vi "Periodic Tasks.vi"(8 "error in":errorcluster) -> ()   [LabVIEW 2014]
doc: "This VI runs in parallel to other tasks. It can contain as many user-defined periodic loops as you need. These can carry out PID or other sorts of timed response."
uses:
  <vilib>/Rock Robotics/WPI/Solenoid/WPI_SolenoidValue.ctl
  teleop_autoFeed.ctl
  <vilib>/Rock Robotics/WPI/CAN/TalonSRX/WPI_CANTalonSRX_APIControlMode.ctl
  <vilib>/Rock Robotics/WPI/CAN/TalonSRX/WPI_CANTalonSRX_Params.ctl
  Robot Global Data.vi
  <vilib>/Rock Robotics/WPI/Solenoid/WPI_SolenoidSetEnum.vi
  <vilib>/Rock Robotics/Network Tables/SD Write Number.vi
  <vilib>/Rock Robotics/WPI/RobotDrive/WPI_RobotDriveGetSetRefNum.vi
  <vilib>/Rock Robotics/WPI/Joystick/WPI_JoystickGetSetRefNum.vi
  <vilib>/Rock Robotics/Network Tables/SD Read Boolean.vi
  <vilib>/Rock Robotics/WPI/RobotDrive/WPI_RobotDriveArcadeDrive_Standard(NoSaturation).vi
  <vilib>/addons/control/pid/pid.llb/PID (DBL).vi
  <vilib>/addons/control/pid/NI_PID_pid.lvlib
panel:
  out "Distance":dbl
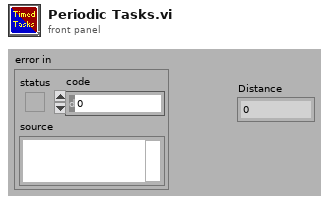
[diagram p1: front panel]
types:
  T1 = typedef "teleop_autoFeed.ctl" = enum16{"wait", "initialize", "arms down 1", "arms open", "arms down 2", "arms close", "up 1st", "back/up"}
  T2 = typedef "WPI_SolenoidValue.ctl" = enum16{"Off", "On", "Forward", "Reverse"}
  T3 = typedef "WPI_SolenoidDevRef.ctl" = cluster{"DevStatus":errorcluster, "Pneumatics Control Module":u8, "Forward Solenoid Channel":T4, "Reverse Solenoid Channel":T4}
  T4 = typedef "WPI_SolenoidChannel.ctl" = enum8{"Solenoid 0", "Solenoid 1", "Solenoid 2", "Solenoid 3", "Solenoid 4", "Solenoid 5", "Solenoid 6", "Solenoid 7", "Invalid"}
  T5 = typedef "WPI_MotorControlDeviceRef.ctl" = cluster{"DeviceStatus":errorcluster, "Type":T6, "PWM":cluster{"Controller":T7, "PWM Channel":T8, "DeadBand":T9}, "CAN":cluster{"Device Number":u8, "Control Mode":T10, "Semaphore":T11, "Max Vout":dbl, "TalonSRX Control Mode":T12}, "Invert":bool, "TransformRef":T13, "InvTransformRef":T13}
  T6 = typedef "WPI_MotorControlType.ctl" = enum16{"PWM", "CAN", "CANTalonSRX"}
  T7 = typedef "FPGA_TypedefDigitalModule.ctl" = enum16{"Controller 1"}
  T8 = typedef "FPGA_DIOPWMChannel.ctl" = enum8{"PWM 0", "PWM 1", "PWM 2", "PWM 3", "PWM 4", "PWM 5", "PWM 6", "PWM 7", "PWM 8", "PWM 9", "PWM MXP 0", "PWM MXP 1", "PWM MXP 2", "PWM MXP 3", "PWM MXP 4", "PWM MXP 5", "PWM MXP 6", "PWM MXP 7", "PWM MXP 8", "PWM MXP 9", "Invalid"}
  T9 = typedef "WPI_PWMDeadband.ctl" = cluster{"Name":string, "maxPositivePwm":i32, "minPositivePwm":i32, "centerPwm":i32, "maxNegativePwm":i32, "minNegativePwm":i32, "angularRange":u16}
  T10 = typedef "WPI_CANJaguar_ControlMode.ctl" = enum8{"Percent VBus", "Current", "Speed", "Position", "Voltage"}
  T11 = typedef "Semaphore RefNum" = refnum<k1>
  T12 = typedef "WPI_CANTalonSRX_APIControlMode.ctl" = enum8{"Percent VBus", "Speed", "Position", "Slave", "Unchanged / Invalid"}
  T13 = typedef "WPI_PWMTransform_ConPane.ctl" = refnum<vi>
  T14 = typedef "WPI_AnalogChannelDevRef.ctl" = cluster{"DevStatus":errorcluster, "Controller":T15, "Analog Channel":T16}
  T15 = typedef "FPGA_TypedefAnalogModule.ctl" = enum16{"Controller 1"}
  T16 = typedef "FPGA_AIChannel.ctl" = enum8{"AI 0", "AI 1", "AI 2", "AI 3", "AI MXP 0", "AI MXP 1", "AI MXP 2", "AI MXP 3", "Invalid"}
  T17 = typedef "WPI_CANTalonSRX_GlobalStatus.ctl" = cluster{"Applied Throttle":dbl, "Module Enabled":bool, "CAN Error":errorcluster, "Closed Loop Error":dbl, "Forward Limit Switch Closed":bool, "Reverse Limit Switch Closed":bool, "Sensor Position":dbl, "Sensor Velocity":dbl, "Current":dbl, "Sticky Fault - Over Temp":bool, "Sticky Fault - Under Voltage":bool, "Sticky Fault - Forward Limit":bool, "Sticky Fault - Reverse Limit":bool, "Sticky Fault - Forward Soft Limit":bool, "Sticky Fault - Reverse Soft Limit":bool, "Brake is Enabled":bool, "Encoder Position":dbl, "Encoder Velocity":dbl, "Encoder Index Count":dbl, "Encoder A Pin State":bool, "Encoder B Pin State":bool, "Encoder Index Pin State":bool, "Analog In":dbl, "Analog In Velocity":dbl, "Temperature (C)":dbl, "Battery Voltage":dbl}
  T18 = typedef "WPI_CANTalonSRX_Params.ctl" = u8
  T19 = typedef "WPI_JoystickDevRef.ctl" = cluster{"Device":T20}
  T20 = typedef "WPI_JoystickDeviceEnum.ctl" = enum16{"USB 0", "USB 1", "USB 2", "USB 3", "USB 4", "USB 5"}
  T21 = typedef "WPI_EncoderDevRef.ctl" = cluster{"DevStatus":errorcluster, "EncoderIndex":T22, "CounterIndex":T23, "DistancePerCount":dbl, "Decoding Type":T24}
  T22 = typedef "FPGA_EncoderIdx.ctl" = enum8{"Enc 0", "Enc 1", "Enc 2", "Enc 3", "Enc 4", "Enc 5", "Enc 6", "Enc 7", "Invalid"}
  T23 = typedef "FPGA_CounterCtrSystemIndex.ctl" = enum8{"Ctr 0", "Ctr 1", "Ctr 2", "Ctr 3", "Ctr 4", "Ctr 5", "Ctr 6", "Ctr 7", "Invalid"}
  T24 = typedef "WPI_EncoderType.ctl" = enum16{"1x", "2x", "4x"}
  T25 = typedef "WPI_RobotDriveDevRef.ctl" = cluster{"DevStatus":errorcluster, "Motors[]":T5[], "Square Inputs":bool, "Max Output":dbl}
  T26 = cluster{"proportional gain (Kc)":dbl, "integral time (Ti, min)":dbl, "derivative time (Td, min)":dbl}
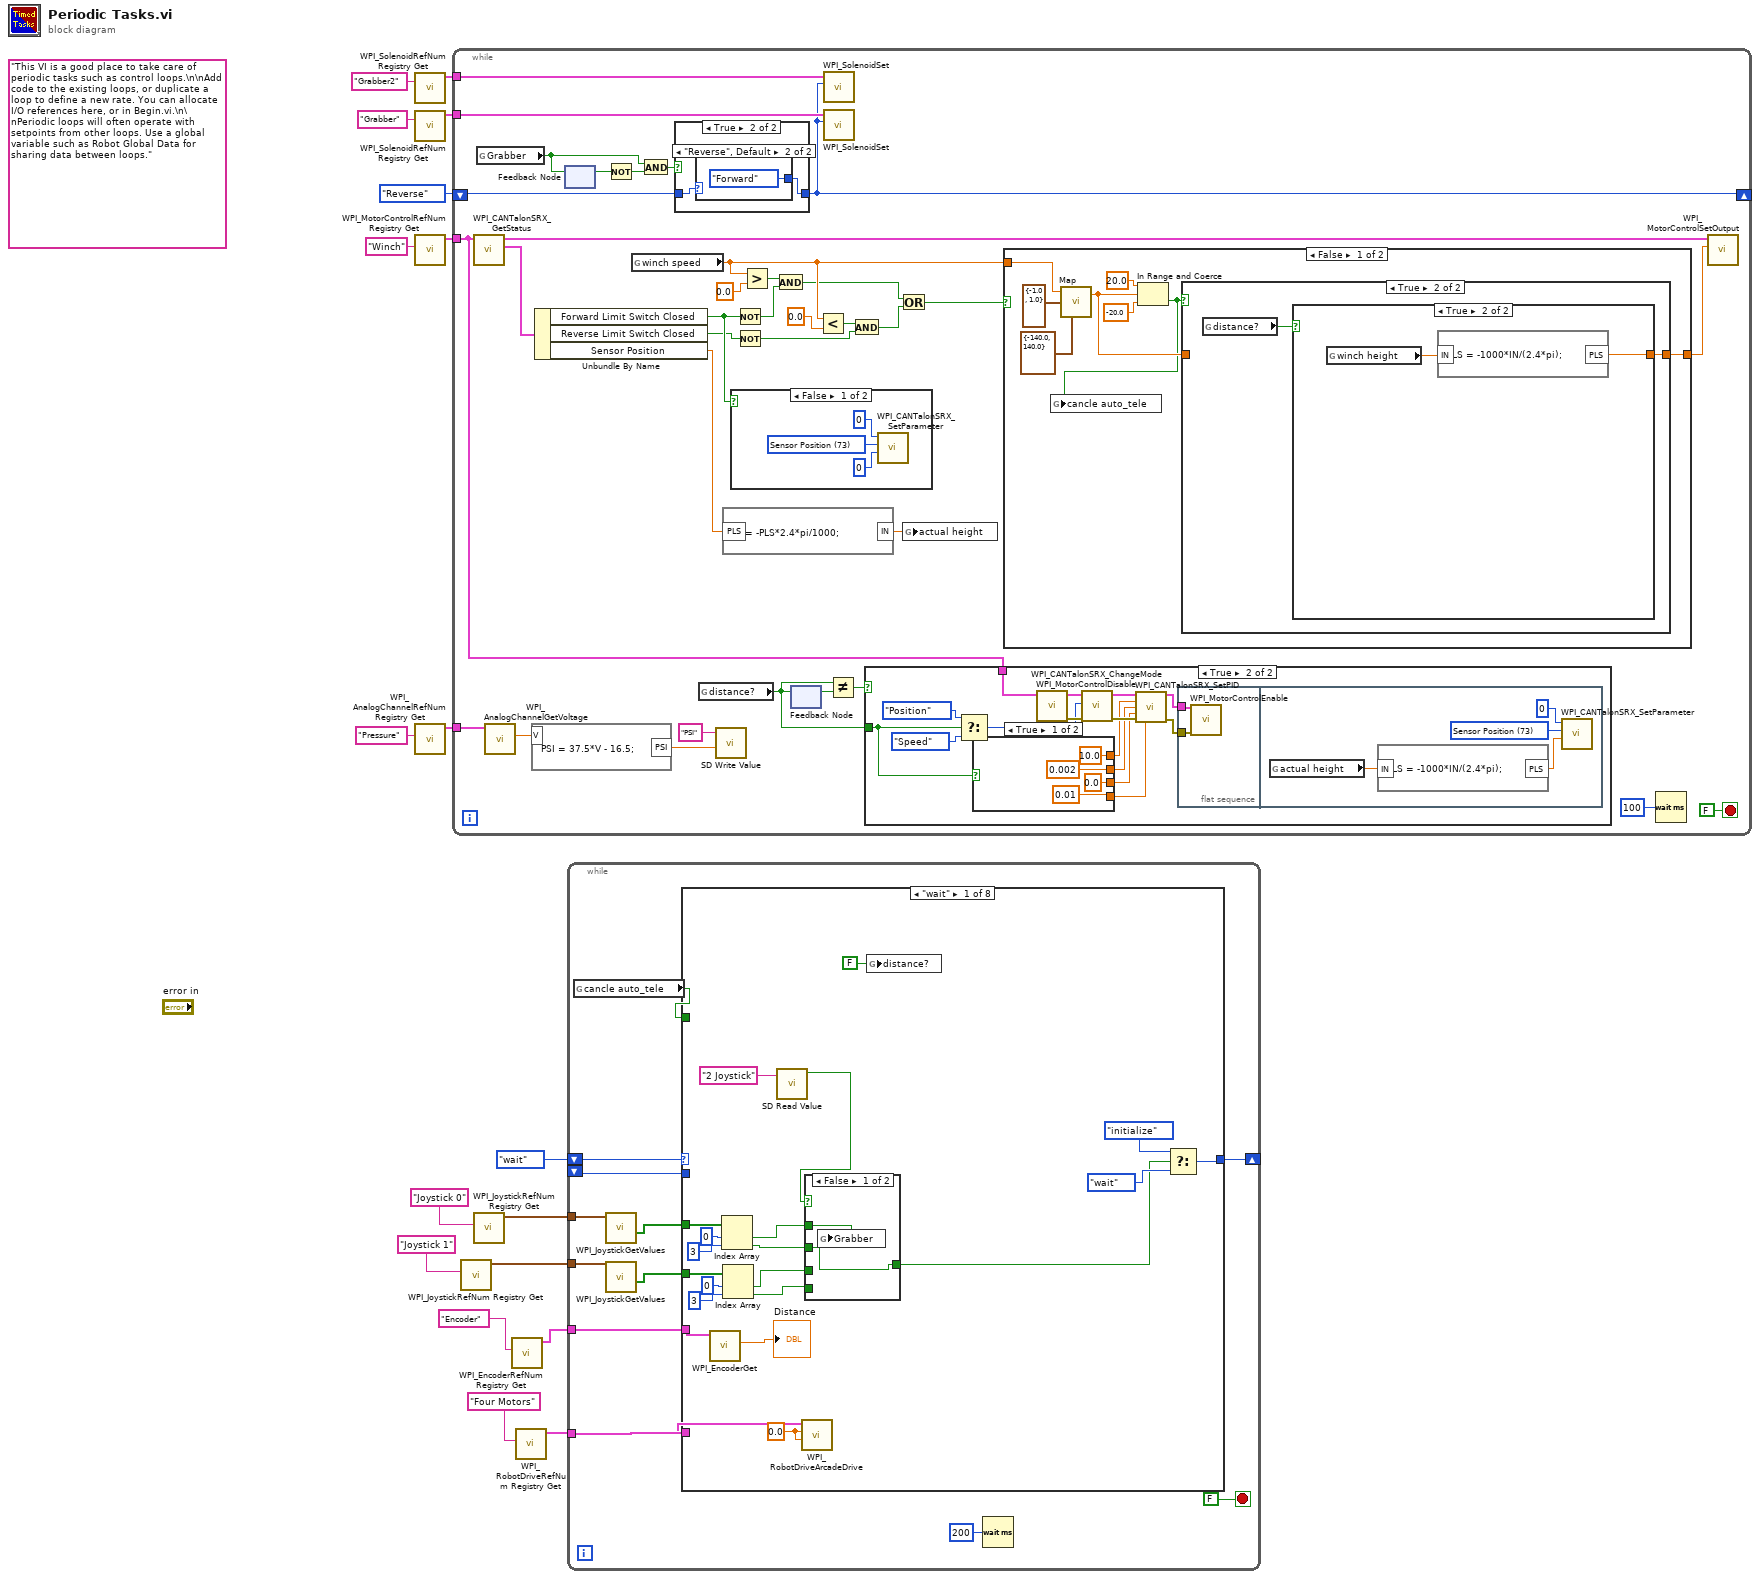
[diagram p0: block diagram]
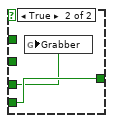
[diagram p2: hidden frame]
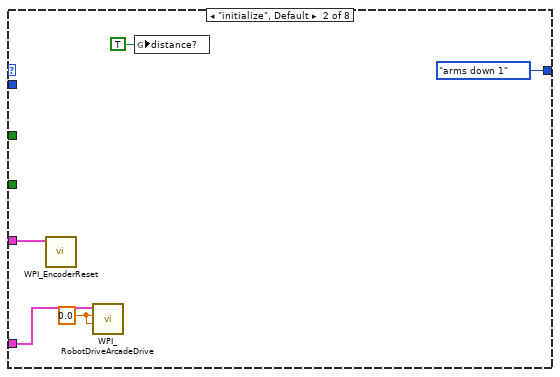
[diagram p3: hidden frame]
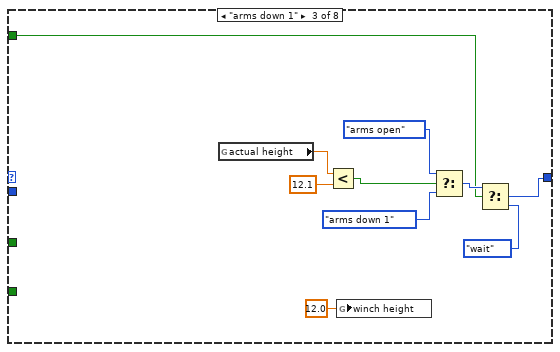
[diagram p4: hidden frame]
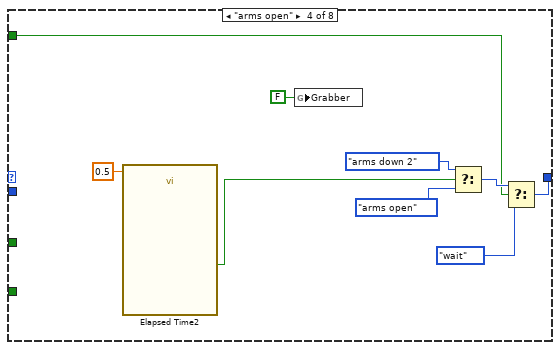
[diagram p5: hidden frame]
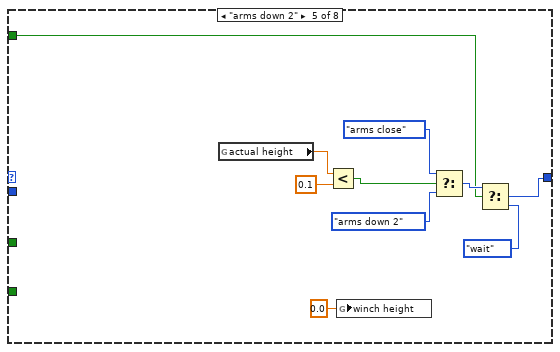
[diagram p6: hidden frame]
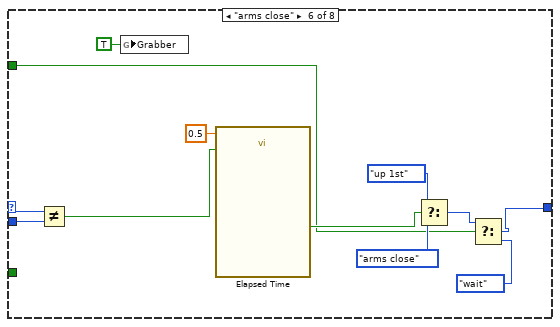
[diagram p7: hidden frame]
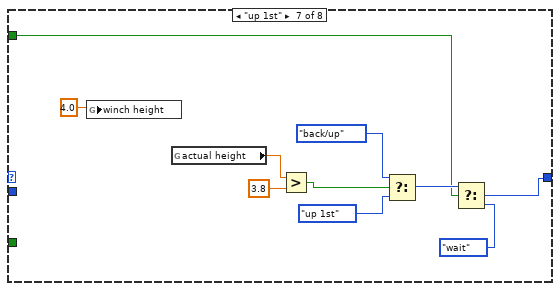
[diagram p8: hidden frame]
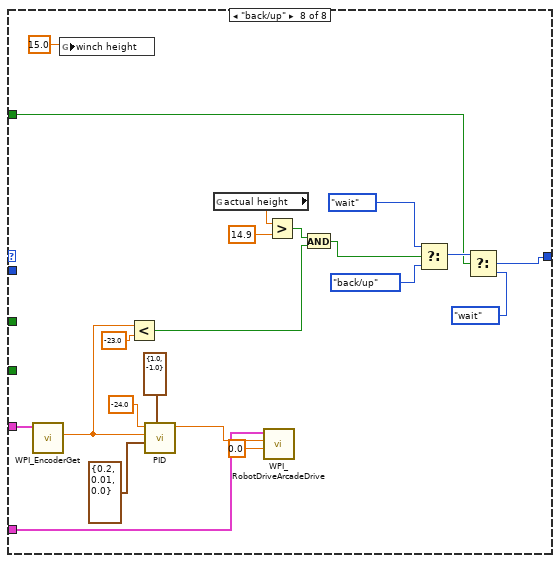
[diagram p9: hidden frame]
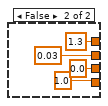
[diagram p11: hidden frame]
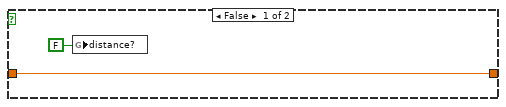
[diagram p13: hidden frame]
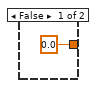
[diagram p14: hidden frame]
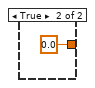
[diagram p15: hidden frame]
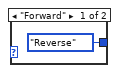
[diagram p17: hidden frame]
diagram:
  w6 = teleop_autoFeed."wait"
  (unwired) "This VI is a good place to take care of periodic tasks such as control loops.\n\nAdd code to the existing loops, or duplicate a loop to define a new rate. You can allocate I/O references here, or in Begin.vi.\n\nPeriodic loops will often operate with setpoints from other loops. Use a global variable such as Robot Global Data for sharing data between loops."
  n1 = call <vilib>:"WPI_SolenoidRefNum Registry Get.vi"("refnum name"="Grabber2") -> ("SolenoidDevRef"=w10:T3)  [unwired: 9 in, 1 out]
  n2 = call <vilib>:"WPI_SolenoidRefNum Registry Get.vi"("refnum name"="Grabber") -> ("SolenoidDevRef"=w16:T3)  [unwired: 9 in, 1 out]
  n3 = call <vilib>:"WPI_MotorControlRefNum Registry Get.vi"("refnum name"="Winch") -> ("MotorControlDevRef"=w14:T5)  [unwired: 9 in, 1 out]
  n4 = call <vilib>:"WPI_AnalogChannelRefNum Registry Get.vi"("refnum name"="Pressure") -> ("AIDeviceRef"=w13:T14)  [unwired: 9 in, 1 out]
  n5 = while {
    tunnel: w16 -> [w48]
    shift-right: [w21] -> _
    shift-left: WPI_SolenoidValue."Reverse" ("Value") -> [w52]
    tunnel: w14 -> [w25]
    tunnel: w13 -> [w44]
    tunnel: w10 -> [w22]
    stop <- FALSE stop-if-true
    n6 = call <vilib>:"WPI_CANTalonSRX_GetStatus.vi"("CAN Talon SRX Ref"=w25) -> ("Talon SRX Status"=w40:T17, "CAN Talon SRX Ref Out"=w29:T5)  [unwired: 8 in, 1 out]
    n7 = global read "Robot Global Data.vi" "Grabber"() -> (w37:bool)
    n8 = call <vilib>:"WPI_AnalogChannelGetVoltage.vi"("AIDeviceRef"=w44) -> ("Voltage"=w47:dbl)  [unwired: 8 in, 2 out]
    n9 = formula code="PSI = 37.5*V - 16.5;"("V"=w47) -> ("PSI"=w46:dbl)
    n10 = Unbundle By Name(w40) -> ("Forward Limit Switch Closed"=w36:bool, "Reverse Limit Switch Closed"=w32:bool, "Sensor Position"=w19:dbl)
    n11 = feedback-in #1(w37) -> ()
    n12 = feedback #1() -> (w49:bool)  [unwired: 1 in]
    n13 = Not(x=w49) -> (.not. x?=w50:bool)
    n14 = global read "Robot Global Data.vi" "winch speed"() -> (w31:dbl)
    n15 = And(x=w37, y=w50) -> (x .and. y?=w51:bool)
    n16 = case shown="True" w51 {
      tunnel: w52 -> [w102 w103]
      tunnel: [w102 w104] -> w21
      frame False {
      }
      frame True {
        n17 = case shown="\"Reverse\", Default" w103 {
          tunnel: [WPI_SolenoidValue."Reverse" ("Value") WPI_SolenoidValue."Forward" ("Value")] -> w104
          frame "Forward" {
          }
          frame "Reverse", Default {
          }
        }
      }
    }
    n18 = global read "Robot Global Data.vi" "distance?"() -> (w26:bool)
    n19 = call-poly <vilib>:"SD Write Value.vi"("Numeric"=w46, "Name"="PSI") -> ()  [unwired: 8 in, 2 out]
    n20 = formula code="IN = -PLS*2.4*pi/1000;"("PLS"=w19) -> ("IN"=w20:dbl)
    n21 = case shown="False" w36 {
      frame False {
        w84 = T18 73 items=["Slot 0 - P"=1, "Slot 0 - I"=2, "Slot 0 - D"=3, "Slot 0 - F"=4, "Slot 0 - I Zone"=5, "Slot 0 - Ramp Rate"=6, "Slot 1 - P"=11, "Slot 1 - I"=12, "Slot 1 - D"=13, "Slot 1 - F"=14, "Slot 1 - I Zone"=15, "Slot 1 - Ramp Rate"=16, "Soft Limit - Forward"=21, "Soft Limit - Reverse"=22, "Soft Limit - Forward Enable"=23, "Soft Limit - Reverse Enable"=24, "On Boot - Brake Mode"=31, "On Boot - Limit Normally Closed - Forward"=32, "On Boot - Limit Normally Closed - Reverse"=33, "On Boot - Limit Disabled - Forward"=34, "On Boot - Limit Disabled - Reverse"=35, "Fault - Over Temp"=41, "Fault - Under Voltage"=42, "Fault - Forward Limit"=43, "Fault - Reverse Limit"=44, "Fault - Hardware Failure"=45, "Fault - Forward Soft Limit"=46, "Fault - Reverse Soft Limit"=47, "Sticky Fault - Over Temp"=48, "Sticky Fault - Under Voltage"=49, "Sticky Fault - Forward Limit"=50, "Sticky Fault - Reverse Limit"=51, "Sticky Fault - Forward Soft Limit"=52, "Sticky Fault - Reverse Soft Limit"=53, "Applied Throttle"=61, "Closed-Loop Error"=62, "Select Feedback Device"=63, "Reverse Closed-Loop Output"=64, "Mode Select"=65, "Profile Slot Select"=66, "Ramp Throttle"=67, "Reverse Feedback Sensor"=68, "Limit Switch Enabled"=69, "Limit Switch Closed - Forward"=70, "Limit Switch Closed - Reverse"=71, "Sensor Position"=73, "Sensor Velocity"=74, "Current"=75, "Brake is Enabled"=76, "Encoder Position"=77, "Encoder Velocity"=78, "Encoder Index Rise Events"=79, "Encoder A Pin State"=80, "Encoder B Pin State"=81, "Encoder Index Pin State"=82, "Analog In with Overflow"=83, "Analog In Velocity"=84, "Temperature"=85, "Battery Voltage"=86, "Reset Count"=87, "Reset Flags"=88, "Firmware Version"=89, "Settings Changed"=90, "Quad Filter Enable"=91, "Ignore Disable Broadcast"=92, "I Accumulator"=93] ("Parameter")
        n22 = call <vilib>:"WPI_CANTalonSRX_SetParameter.vi"("Value"=0, "Parameter"=w84, "Device ID (0)"=u8 0) -> ()  [unwired: 7 in, 2 out]
      }
      frame True {
      }
    }
    n23 = Not(x=w36) -> (.not. x?=w38:bool)
    n24 = Not(x=w32) -> (.not. x?=w35:bool)
    n25 = Greater?(x=w31, y=0.0) -> (0:w39:bool)
    n26 = And(x=w39, y=w38) -> (x .and. y?=w24:bool)
    n27 = feedback-in #2(w26) -> ()
    n28 = feedback #2() -> (w28:bool)  [unwired: 1 in]
    n29 = Less?(x=w31, y=0.0) -> (x < y?=w34:bool)
    n30 = call-poly <vilib>:"WPI_SolenoidSet.vi"("Value"=w21, "SolenoidDevRef"=w22) -> ()  [unwired: 8 in, 2 out]
    n31 = call-poly <vilib>:"WPI_SolenoidSet.vi"("Value"=w21, "SolenoidDevRef"=w48) -> ()  [unwired: 8 in, 2 out]
    n32 = Not Equal?(x=w26, y=w28) -> (x != y?=w27:bool)
    n33 = And(x=w34, y=w35) -> (x .and. y?=w30:bool)
    n34 = case shown="True" w27 {
      tunnel: w26 -> [_ w58]
      tunnel: w25 -> [_ w54]
      frame False {
      }
      frame True {
        n35 = Select(t=WPI_CANTalonSRX_APIControlMode."Position" ("Control Mode"), s=w58, f=WPI_CANTalonSRX_APIControlMode."Speed") -> (s? t:f=w55:T12)
        n36 = case shown="True" w58 {
          tunnel: [10.0 1.3] -> w62
          tunnel: [0.002 0.03] -> w61
          tunnel: [0.0 0.0] -> w60
          tunnel: [0.01 1.0] -> w59
          frame True {
          }
          frame False {
          }
        }
        n37 = call <vilib>:"WPI_MotorControlDisable.vi"("MotorControlDevRef"=w54) -> ("error out"=w57:errorcluster, "MotorControlDevRef"=w56:T5)  [unwired: 9 in]
        n38 = call <vilib>:"WPI_CANTalonSRX_ChangeMode.vi"("error in (no error)"=w57, "Control Mode"=w55, "CAN Talon SRX Ref"=w56) -> ("error out"=w65:errorcluster, "CAN Talon SRX Ref Out"=w66:T5)  [unwired: 7 in]
        n39 = call <vilib>:"WPI_CANTalonSRX_SetPID.vi"("CAN Talon SRX Ref"=w66, "P"=w62, "I"=w61, "D"=w60, "error in (no error)"=w65, "F"=w59) -> ("CAN Talon SRX Ref Out"=w64:T5, "error out"=w63:errorcluster)  [unwired: 8 in]
        n40 = flat-sequence {
          tunnel: w64 -> [w70]
          tunnel: w63 -> [w69]
          frame #0 {
            n41 = call <vilib>:"WPI_MotorControlEnable.vi"("error in (no error)"=w69, "CAN Jaguar Ref"=w70) -> ()  [unwired: 8 in, 2 out]
          }
          frame #1 {
            w72 = T18 73 items=["Slot 0 - P"=1, "Slot 0 - I"=2, "Slot 0 - D"=3, "Slot 0 - F"=4, "Slot 0 - I Zone"=5, "Slot 0 - Ramp Rate"=6, "Slot 1 - P"=11, "Slot 1 - I"=12, "Slot 1 - D"=13, "Slot 1 - F"=14, "Slot 1 - I Zone"=15, "Slot 1 - Ramp Rate"=16, "Soft Limit - Forward"=21, "Soft Limit - Reverse"=22, "Soft Limit - Forward Enable"=23, "Soft Limit - Reverse Enable"=24, "On Boot - Brake Mode"=31, "On Boot - Limit Normally Closed - Forward"=32, "On Boot - Limit Normally Closed - Reverse"=33, "On Boot - Limit Disabled - Forward"=34, "On Boot - Limit Disabled - Reverse"=35, "Fault - Over Temp"=41, "Fault - Under Voltage"=42, "Fault - Forward Limit"=43, "Fault - Reverse Limit"=44, "Fault - Hardware Failure"=45, "Fault - Forward Soft Limit"=46, "Fault - Reverse Soft Limit"=47, "Sticky Fault - Over Temp"=48, "Sticky Fault - Under Voltage"=49, "Sticky Fault - Forward Limit"=50, "Sticky Fault - Reverse Limit"=51, "Sticky Fault - Forward Soft Limit"=52, "Sticky Fault - Reverse Soft Limit"=53, "Applied Throttle"=61, "Closed-Loop Error"=62, "Select Feedback Device"=63, "Reverse Closed-Loop Output"=64, "Mode Select"=65, "Profile Slot Select"=66, "Ramp Throttle"=67, "Reverse Feedback Sensor"=68, "Limit Switch Enabled"=69, "Limit Switch Closed - Forward"=70, "Limit Switch Closed - Reverse"=71, "Sensor Position"=73, "Sensor Velocity"=74, "Current"=75, "Brake is Enabled"=76, "Encoder Position"=77, "Encoder Velocity"=78, "Encoder Index Rise Events"=79, "Encoder A Pin State"=80, "Encoder B Pin State"=81, "Encoder Index Pin State"=82, "Analog In with Overflow"=83, "Analog In Velocity"=84, "Temperature"=85, "Battery Voltage"=86, "Reset Count"=87, "Reset Flags"=88, "Firmware Version"=89, "Settings Changed"=90, "Quad Filter Enable"=91, "Ignore Disable Broadcast"=92, "I Accumulator"=93] ("Parameter")
            n42 = global read "Robot Global Data.vi" "actual height"() -> (w71:dbl)
            n43 = formula code="PLS = -1000*IN/(2.4*pi);"("IN"=w71) -> ("PLS"=w74:dbl)
            n44 = call <vilib>:"WPI_CANTalonSRX_SetParameter.vi"("Value"=w74, "Parameter"=w72, "Device ID (0)"=u8 0) -> ()  [unwired: 7 in, 2 out]
          }
        }
      }
    }
    n45 = Or(x=w24, y=w30) -> (x .or. y?=w23:bool)
    n46 = global write "Robot Global Data.vi" "actual height"(w20) -> ()
    n47 = case shown="False" w23 {
      tunnel: [w93 0.0 ("Output")] -> w43
      tunnel: w31 -> [w87 _]
      frame False {
        n48 = call "Map.vi"("Input"=w87, "Input range"=cluster{"Min":dbl, "Max":dbl} {"Min"=-1.0, "Max"=1.0}, "Output range"=cluster{"Min":dbl, "Max":dbl} {"Min"=-140.0, "Max"=140.0}) -> ("Output"=w88:dbl)  [unwired: 3 in]
        n49 = In Range and Coerce(upper limit=20.0, x=w88, lower limit=-20.0) -> (In Range?=w86:bool)  [unwired: 1 out]
        n50 = global write "Robot Global Data.vi" "cancle auto_tele"(w86) -> ()
        n51 = case shown="True" w86 {
          tunnel: w88 -> [w95 _]
          tunnel: [w95 w96] -> w93
          frame False {
            n52 = global write "Robot Global Data.vi" "distance?"(FALSE ("distance?")) -> ()
          }
          frame True {
            n53 = global read "Robot Global Data.vi" "distance?"() -> (w97:bool)
            n54 = case shown="True" w97 {
              tunnel: [0.0 w100] -> w96
              frame False {
              }
              frame True {
                n55 = global read "Robot Global Data.vi" "winch height"() -> (w99:dbl)
                n56 = formula code="PLS = -1000*IN/(2.4*pi);"("IN"=w99) -> ("PLS"=w100:dbl)
              }
            }
          }
        }
      }
      frame True {
      }
    }
    n57 = Wait (ms)(milliseconds to wait=u32 100) -> ()  [unwired: 1 out]
    n58 = call <vilib>:"WPI_MotorControlSetOutput.vi"("Output"=w43, "MotorControlDevRef"=w29) -> ()  [unwired: 7 in, 3 out]
  }
  n59 = call <vilib>:"WPI_JoystickRefNum Registry Get.vi"("refnum name"="Joystick 1") -> ("JoystickDevRef"=w1:T19)  [unwired: 1 in, 9 out]
  n60 = call <vilib>:"WPI_JoystickRefNum Registry Get.vi"("refnum name"="Joystick 0") -> ("JoystickDevRef"=w3:T19)  [unwired: 1 in, 9 out]
  n61 = call <vilib>:"WPI_EncoderRefNum Registry Get.vi"("refnum name"="Encoder") -> ("EncoderDevRef"=w4:T21)  [unwired: 9 in, 1 out]
  n62 = call <vilib>:"WPI_RobotDriveRefNum Registry Get.vi"("refnum name"="Four Motors") -> ("RobotDriveDevRef"=w8:T25)  [unwired: 9 in, 1 out]
  n63 = while {
    shift-right: [w115] -> _
    shift-left: w6 -> [w117]
    tunnel: w8 -> [w116]
    shift-left: w6 -> [w114]
    tunnel: w4 -> [w113]
    tunnel: w3 -> [w112]
    tunnel: w1 -> [w109]
    stop <- FALSE stop-if-true
    n64 = global read "Robot Global Data.vi" "cancle auto_tele"() -> (w107:bool)
    n65 = call <vilib>:"WPI_JoystickGetValues.vi"("JoystickDevRef"=w112) -> ("Buttons"=w111:bool[])  [unwired: 6 in, 4 out]
    n66 = call <vilib>:"WPI_JoystickGetValues.vi"("JoystickDevRef"=w109) -> ("Buttons"=w108:bool[])  [unwired: 6 in, 4 out]
    n67 = case shown="\"wait\"" w117 {
      selector: w117 -> [_ _ _ _ _ w188 _ _]
      tunnel: w116 -> [w130 w148 _ _ _ _ _ w211]
      tunnel: [w134 teleop_autoFeed."arms down 1" w151 w164 w170 w180 w192 w202] -> w115
      tunnel: w111 -> [w138 _ _ _ _ _ _ _]
      tunnel: w114 -> [_ _ _ _ _ w187 _ _]
      tunnel: w113 -> [w129 w144 _ _ _ _ _ w215]
      tunnel: w108 -> [w125 _ _ _ _ _ _ _]
      tunnel: w107 -> [_ _ w149 w161 w168 w178 w190 w200]
      frame "wait" {
        w131 = 0.0 ("X axis value")
        n68 = call <vilib>:"WPI_EncoderGet.vi"("EncoderDevRef"=w129) -> ("Distance"=→"Distance":dbl)  [unwired: 5 in, 5 out]
        n69 = Index Array(array=w138, index #1=0 ("index"), index #2=3 ("index")) -> (element #1=w137:bool, element #2=w122:bool)
        n70 = Index Array(array=w125, index #1=0 ("index"), index #2=3 ("index")) -> (element #1=w120:bool, element #2=w119:bool)
        n71 = call-poly <vilib>:"SD Read Value.vi"("Name"="2 Joystick") -> ("Boolean"=w123:bool)  [unwired: 8 in, 2 out]
        n72 = call-poly <vilib>:"WPI_RobotDriveArcadeDrive.vi"("Y axis value"=w131, "X axis value"=w131, "RobotDriveDevRef"=w130) -> ()  [unwired: 6 in, 3 out]
        n73 = case shown="False" w123 {
          tunnel: w137 -> [w141 _]
          tunnel: w122 -> [w140 _]
          tunnel: [w140 w143] -> w121
          tunnel: w120 -> [_ w142]
          tunnel: w119 -> [_ w143]
          frame False {
            n74 = global write "Robot Global Data.vi" "Grabber"(w141) -> ()
          }
          frame True {
            n75 = global write "Robot Global Data.vi" "Grabber"(w142) -> ()
          }
        }
        n76 = global write "Robot Global Data.vi" "distance?"(FALSE ("distance?")) -> ()
        n77 = Select(t=teleop_autoFeed."initialize", s=w121, f=teleop_autoFeed."wait") -> (s? t:f=w134:T1)
      }
      frame "initialize", Default {
        w147 = 0.0 ("X axis value")
        n78 = call <vilib>:"WPI_EncoderReset.vi"("EncoderDevRef"=w144) -> ()  [unwired: 9 in, 2 out]
        n79 = call-poly <vilib>:"WPI_RobotDriveArcadeDrive.vi"("Y axis value"=w147, "X axis value"=w147, "RobotDriveDevRef"=w148) -> ()  [unwired: 6 in, 3 out]
        n80 = global write "Robot Global Data.vi" "distance?"(TRUE ("distance?")) -> ()
      }
      frame "arms down 1" {
        n81 = global read "Robot Global Data.vi" "actual height"() -> (w155:dbl)
        n82 = Less?(x=w155, y=12.1) -> (x < y?=w153:bool)
        n83 = global write "Robot Global Data.vi" "winch height"(12.0 ("winch height")) -> ()
        n84 = Select(t=teleop_autoFeed."arms open", s=w153, f=teleop_autoFeed."arms down 1") -> (s? t:f=w152:T1)
        n85 = Select(t=w152, s=w149, f=teleop_autoFeed."wait") -> (s? t:f=w151:T1)
      }
      frame "arms open" {
        n86 = call "Elapsed Time2"("Time Target (s)"=0.5) -> ("Time has Elapsed"=w159:bool)  [unwired: 11 in, 7 out]
        n87 = global write "Robot Global Data.vi" "Grabber"(FALSE ("Grabber")) -> ()
        n88 = Select(t=teleop_autoFeed."arms down 2", s=w159, f=teleop_autoFeed."arms open") -> (s? t:f=w163:T1)
        n89 = Select(t=w163, s=w161, f=teleop_autoFeed."wait") -> (s? t:f=w164:T1)
      }
      frame "arms down 2" {
        n90 = global read "Robot Global Data.vi" "actual height"() -> (w174:dbl)
        n91 = Less?(x=w174, y=0.1) -> (x < y?=w172:bool)
        n92 = global write "Robot Global Data.vi" "winch height"(0.0 ("winch height")) -> ()
        n93 = Select(t=teleop_autoFeed."arms close", s=w172, f=teleop_autoFeed."arms down 2") -> (s? t:f=w171:T1)
        n94 = Select(t=w171, s=w168, f=teleop_autoFeed."wait") -> (s? t:f=w170:T1)
      }
      frame "arms close" {
        n95 = Not Equal?(x=w188, y=w187) -> (x != y?=w186:bool)
        n96 = global write "Robot Global Data.vi" "Grabber"(TRUE ("Grabber")) -> ()
        n97 = call "Elapsed Time"("Time Target (s)"=0.5, "Reset"=w186) -> ("Time has Elapsed"=w184:bool)  [unwired: 10 in, 7 out]
        n98 = Select(t=teleop_autoFeed."up 1st", s=w184, f=teleop_autoFeed."arms close") -> (s? t:f=w179:T1)
        n99 = Select(t=w179, s=w178, f=teleop_autoFeed."wait") -> (s? t:f=w180:T1)
      }
      frame "up 1st" {
        n100 = global write "Robot Global Data.vi" "winch height"(4.0 ("winch height")) -> ()
        n101 = global read "Robot Global Data.vi" "actual height"() -> (w196:dbl)
        n102 = Greater?(x=w196, y=3.8) -> (0:w194:bool)
        n103 = Select(t=teleop_autoFeed."back/up", s=w194, f=teleop_autoFeed."up 1st") -> (s? t:f=w191:T1)
        n104 = Select(t=w191, s=w190, f=teleop_autoFeed."wait") -> (s? t:f=w192:T1)
      }
      frame "back/up" {
        n105 = call <vilib>:"WPI_EncoderGet.vi"("EncoderDevRef"=w215) -> ("Distance"=w209:dbl)  [unwired: 5 in, 5 out]
        n106 = global write "Robot Global Data.vi" "winch height"(15.0 ("winch height")) -> ()
        n107 = Less?(x=w209, y=-23.0) -> (x < y?=w207:bool)
        n108 = call-poly <vilib>:"PID.vi"("output range"=cluster{"output high":dbl, "output low":dbl} {"output high"=1.0, "output low"=-1.0}, "PID gains"=T26 {"proportional gain (Kc)"=0.2, "integral time (Ti, min)"=0.01, "derivative time (Td, min)"=0.0}, "process variable"=w209, "setpoint"=-24.0) -> ("output"=w210:dbl)  [unwired: 6 in, 1 out]
        n109 = global read "Robot Global Data.vi" "actual height"() -> (w217:dbl)
        n110 = call-poly <vilib>:"WPI_RobotDriveArcadeDrive.vi"("Y axis value"=0.0, "X axis value"=w210, "RobotDriveDevRef"=w211) -> ()  [unwired: 6 in, 3 out]
        n111 = Greater?(x=w217, y=14.9) -> (0:w206:bool)
        n112 = And(x=w206, y=w207) -> (x .and. y?=w205:bool)
        n113 = Select(t=teleop_autoFeed."wait", s=w205, f=teleop_autoFeed."back/up") -> (s? t:f=w201:T1)
        n114 = Select(t=w201, s=w200, f=teleop_autoFeed."wait") -> (s? t:f=w202:T1)
      }
    }
    n115 = Wait (ms)(milliseconds to wait=u32 200) -> ()  [unwired: 1 out]
  }
